vi "PhantomDisplacementSensor.vi"() -> ()   [LabVIEW 2011]
panel:
  in  "nominal radius":dbl=12.5
  in  "Enable chart":bool
  out "Waveform Chart":dbl(graph)
  in  "out of center y":dbl=0.01
  in  "out of center x":dbl=0.1
  in  "frequency":dbl=3.2
  in  "waviness":dbl=0.005
  in  "noise":dbl=0.0015
  in  "stop":bool
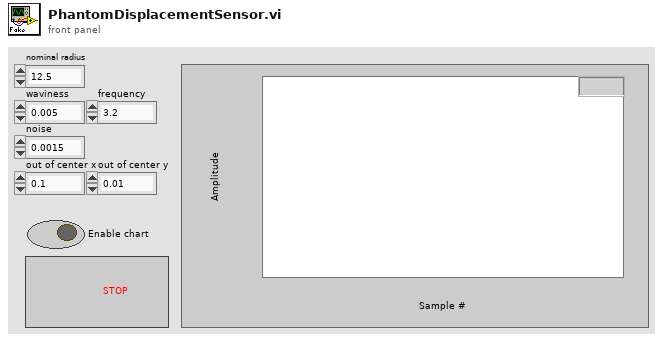
[diagram p1: front panel]
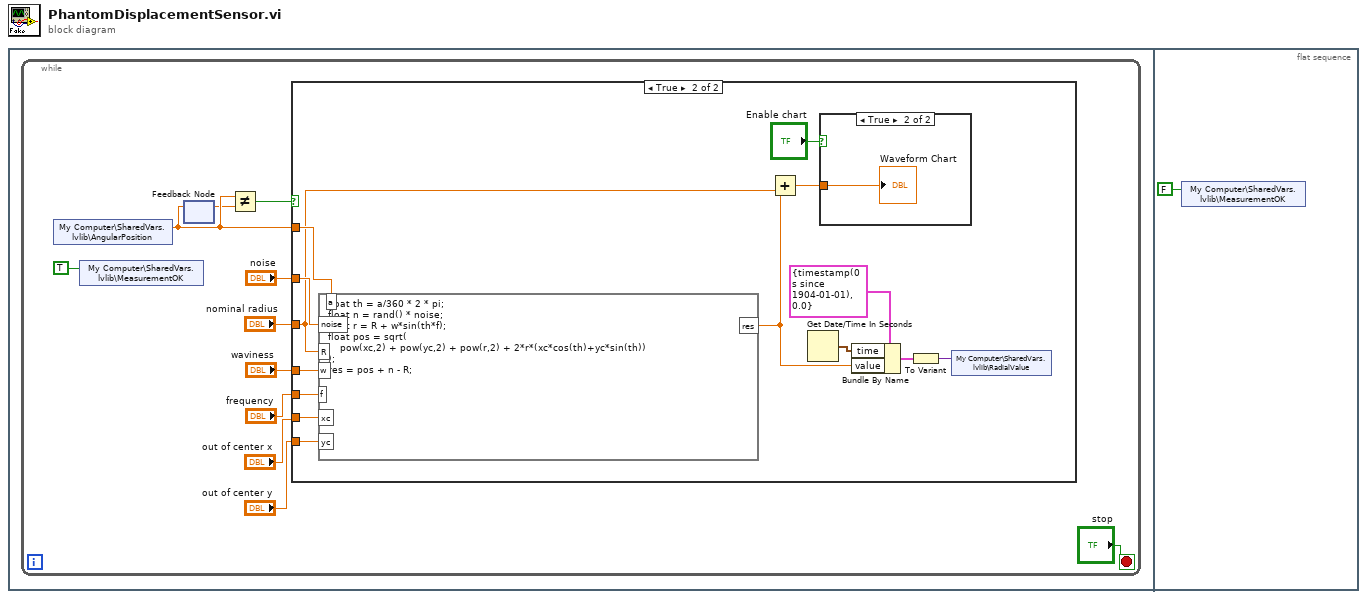
[diagram p0: block diagram]
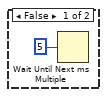
[diagram p2: hidden frame]
diagram:
  n1 = flat-sequence {
    frame #0 {
      n2 = while {
        stop <- "stop" stop-if-true
        n3 = shared-variable "My Computer\\SharedVars.lvlib\\AngularPosition"() -> (w10:dbl)  [unwired: 1 in, 1 out]
        n4 = shared-variable "My Computer\\SharedVars.lvlib\\MeasurementOK"(TRUE ("MeasurementOK")) -> ()  [unwired: 1 in, 1 out]
        n5 = feedback-in #1(w10) -> ()
        n6 = feedback #1() -> (w8:dbl)  [unwired: 1 in]
        n7 = Not Equal?(x=w10, y=w8) -> (x != y?=w9:bool)
        n8 = case shown="True" w9 {
          tunnel: w10 -> [_ w26]
          tunnel: "noise" -> [_ w21]
          tunnel: "waviness" -> [_ w20]
          tunnel: "frequency" -> [_ w19]
          tunnel: "out of center x" -> [_ w18]
          tunnel: "out of center y" -> [_ w17]
          tunnel: "nominal radius" -> [_ w15]
          frame False {
            n9 = Wait Until Next ms Multiple(millisecond multiple=u32 5) -> ()  [unwired: 1 out]
          }
          frame True {
            n10 = formula code="float th = a/360 * 2 * pi;\nfloat n = rand() * noise;\nfloat r = R + w*sin(th*f);\nfloat pos = sqrt( \n    pow(xc,2) + pow(yc,2) + pow(r,2) + 2*r*(xc*cos(th)+yc*sin(th))\n);\nres = pos + n - R;"("a"=w26, "noise"=w21, "f"=w19, "xc"=w18, "yc"=w17, "w"=w20, "R"=w15) -> ("res"=w14:dbl)
            n11 = Add(x=w14, y=w15) -> (x+y=w13:dbl)
            n12 = Get Date/Time In Seconds() -> (seconds since 1Jan1904=w25:timestamp)
            n13 = case shown="True" "Enable chart" {
              tunnel: w13 -> [_ w27]
              frame False {
              }
              frame True {
                "Waveform Chart" <- w27
              }
            }
            n14 = Bundle By Name(cluster=cluster{"time":timestamp, "value":dbl} {"time"=timestamp(0 s since 1904-01-01), "value"=0.0} ("input cluster"), "time"=w25, "value"=w14) -> (w23:cluster{"time":timestamp, "value":dbl})
            n15 = To Variant(anything=w23) -> (Variant=w22:variant)
            n16 = shared-variable "My Computer\\SharedVars.lvlib\\RadialValue"(w22) -> ()  [unwired: 1 in, 1 out]
          }
        }
      }
    }
    frame #1 {
      n17 = shared-variable "My Computer\\SharedVars.lvlib\\MeasurementOK"(FALSE ("MeasurementOK")) -> ()  [unwired: 1 in, 1 out]
    }
  }
